vi "Completed.vi"(8 "error in (no error)":errorcluster, 11 "Instruction in":refnum<class "Instruction.lvclass">) -> (0 "error out":errorcluster, 3 "Completed":bool)   [LabVIEW 2015, in "Instruction.lvclass"]
uses:
  Instruction.lvclass
  MovementInstruction.lvclass
  TurnInstruction.lvclass
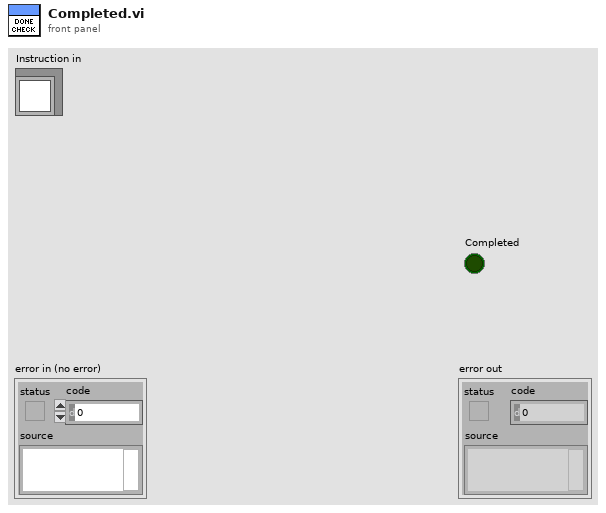
[diagram p1: front panel]
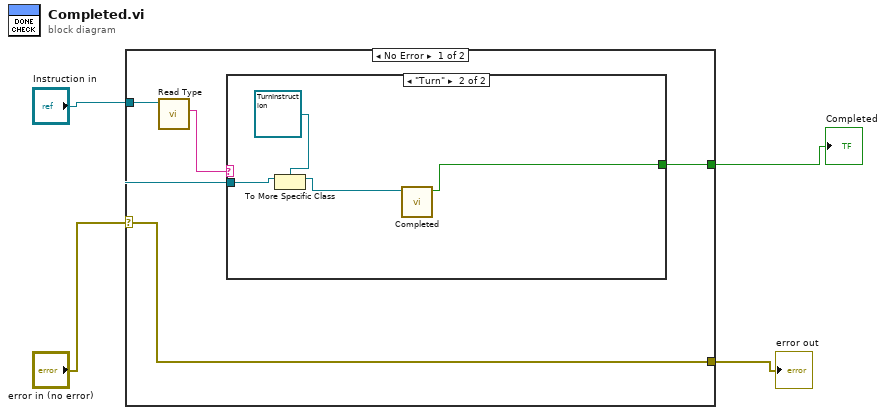
[diagram p0: block diagram]
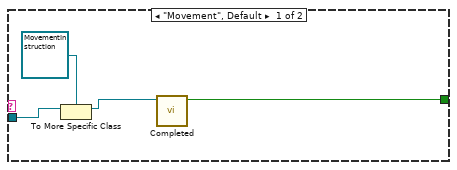
[diagram p2: hidden frame]
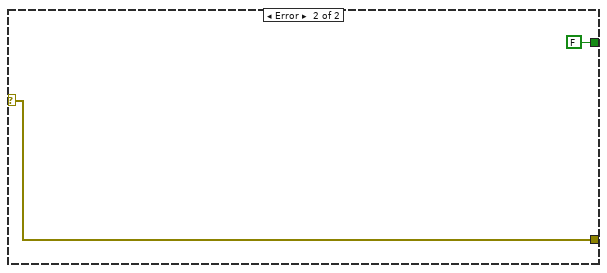
[diagram p3: hidden frame]
diagram:
  n1 = case shown="No Error" "error in (no error)" {
    selector: "error in (no error)" -> [w5 w18]
    tunnel: "Instruction in" -> [w7 _]
    tunnel: [w6 FALSE ("Completed")] -> w3
    tunnel: [w5 w18] -> w1
    frame No Error {
      n2 = call-dynamic "Read Type.vi"("Instruction in"=w7) -> ("Type"=w8:string)  [unwired: 8 in, 2 out]
      n3 = case shown="\"Turn\"" w8 {
        tunnel: w7 -> [w11 w16]
        tunnel: [w9 w13] -> w6
        frame "Movement", Default {
          n4 = To More Specific Class(target class=refnum<class "MovementInstruction.lvclass"> refnum ("MovementInstruction.lvclass"), reference=w11) -> (specific class reference=w10:refnum<class "MovementInstruction.lvclass">)  [unwired: 1 in, 1 out]
          n5 = call-dynamic "Completed.vi"("MovementInstruction.lvclass 2"=w10) -> ("Completed"=w9:bool)  [unwired: 9 in, 1 out]
        }
        frame "Turn" {
          n6 = To More Specific Class(target class=refnum<class "TurnInstruction.lvclass"> refnum ("TurnInstruction.lvclass"), reference=w16) -> (specific class reference=w14:refnum<class "TurnInstruction.lvclass">)  [unwired: 1 in, 1 out]
          n7 = call-dynamic "Completed.vi"("TurnInstruction.lvclass"=w14) -> ("Completed"=w13:bool)  [unwired: 9 in, 1 out]
        }
      }
    }
    frame Error {
    }
  }
  "error out" <- w1
  "Completed" <- w3
